vi "Bore pos (SubVI).vi"(0 "Position.":dbl format="%#_13g") -> (1 "Duty":dbl, 2 "freq [Hz]":dbl=50.0)   [LabVIEW 2018]
panel:
  out "offset [%FS]":dbl
  in  "null offset":bool
  # "Value (-180 to 180)"
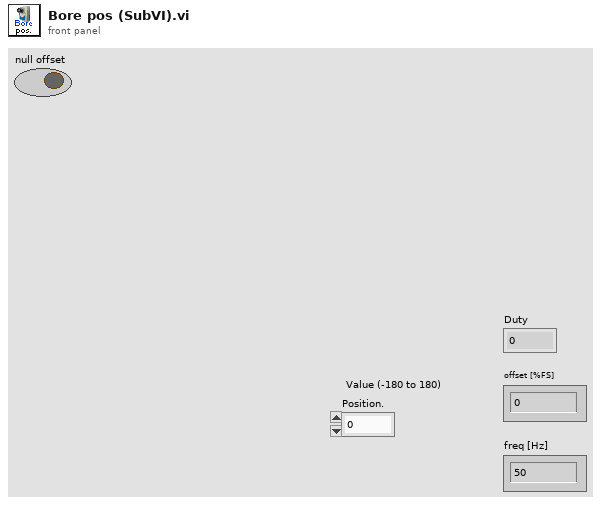
[diagram p1: front panel]
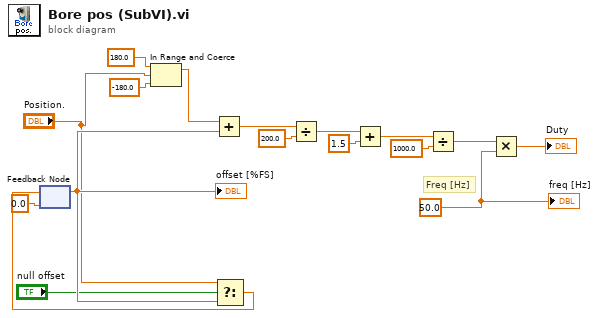
[diagram p0: block diagram]
diagram:
  w10 = 50.0 ("freq [Hz]")
  # "Freq [Hz]"
  n1 = feedback #1(0.0 ("position [%FS]")) -> (w14:dbl)
  "offset [%FS]" <- w14
  n2 = In Range and Coerce(upper limit=180.0, x="Position.", lower limit=-180.0 ("upper limit")) -> (coerced(x)=w1:dbl)  [unwired: 1 out]
  n3 = Add(x=w1, y=w14) -> (x+y=w13:dbl)
  n4 = Select(t="Position.", s="null offset", f=w14) -> (s? t:f=w12:dbl)
  n5 = feedback-in #1(w12) -> ()
  n6 = Divide(x=w13, y=200.0) -> (x/y=w6:dbl)
  n7 = Add(x=w6, y=1.5) -> (x+y=w8:dbl)
  n8 = Divide(x=w8, y=1000.0) -> (x/y=w15:dbl)
  n9 = Multiply(x=w15, y=w10) -> (x*y=→"Duty":dbl)
  "freq [Hz]" <- w10
